vi "SubVI_ReadArray.vi"(2 "Path":path) -> (0 "Array":dbl[](array[numeric]))   [LabVIEW 2018]
panel:
  in  "Data Type":dbl[](array[numeric])
  out "error out":errorcluster
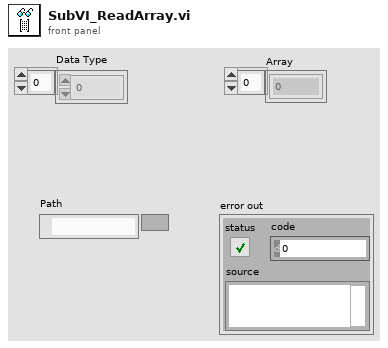
[diagram p1: front panel]
types:
  T1 = enum16{"open", "replace", "create", "open or create", "replace or create", "replace or create with confirmation"}
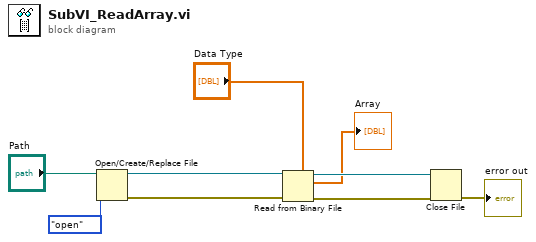
[diagram p0: block diagram]
diagram:
  n1 = Open/Create/Replace File(file path (use dialog)="Path", operation (0:open)=T1."open") -> (refnum out=w6:refnum<file>, error out=w5:errorcluster)  [unwired: 4 in, 1 out]
  n2 = Read from Binary File(5:"Data Type", 8:w5, 11:w6) -> (0:w4:errorcluster, 2:→"Array":dbl[], 3:w3:refnum<file>)  [unwired: 3 in, 1 out]
  n3 = Close File(refnum=w3, error in=w4) -> (error out=→"error out":errorcluster)  [unwired: 1 out]
